vi "Get LVObjectArray.vi"(8 "error in (no error)":errorcluster, 11 "LVObjectArrayMsg in":refnum<class "LVObjectArrayMsg.lvclass">) -> (0 "error out":errorcluster, 2 "Message Data":refnum<class>[](array[class]), 3 "LVObjectArrayMsg out":refnum<class "LVObjectArrayMsg.lvclass">)   [LabVIEW 2018, in "LapDog.Messaging.v3.NativeArrays.lvlib" / "LVObjectArrayMsg.lvclass"]
doc: "Returns the data contained in the message.\n\nThis method executes regardless of the error in state."
uses:
  LVObjectArrayMsg.lvclass
  LVObjectArrayMsg.lvclass/LVObjectArrayMsg.ctl
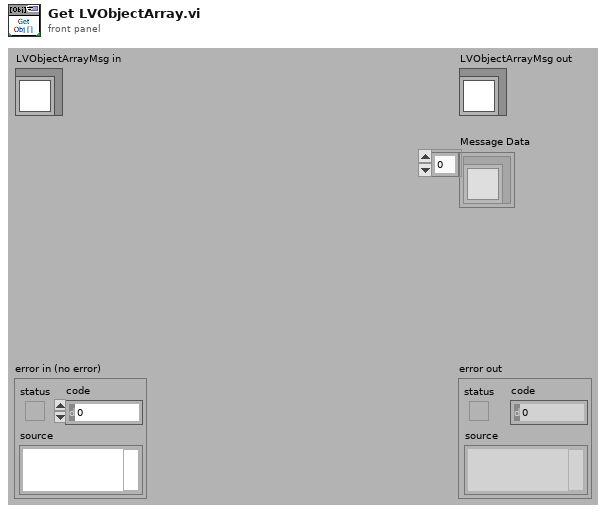
[diagram p1: front panel]
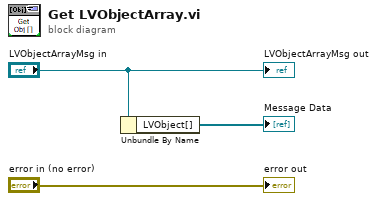
[diagram p0: block diagram]
diagram:
  n1 = Unbundle By Name("LVObjectArrayMsg in") -> ("LVObject[]"=→"Message Data":refnum<class>[])
  "error out" <- "error in (no error)"
  "LVObjectArrayMsg out" <- "LVObjectArrayMsg in"
